vi "(Pop-up) Header Make.vi"(7 "IN Info":string, 8 "error in (no error)":errorcluster caption="에러 입력(에러 없음)", 9 "IN RB/GB":bool, 10 "IN Current Limit":dbl format="%.2f mA", 11 "IN Taget Voltage":dbl format="%.1f V") -> (0 "error out":errorcluster caption="에러 출력", 1 "Start":bool, 2 "Out Start Delay":dbl format="%<%H:%M:%S>t")   [LabVIEW 2017]
uses:
  <vilib>/Utility/miscctls.llb/LVPointTypeDef.ctl
panel:
  in  "Start Delay":dbl format="%<%H:%M:%S>t"
  out "RB/GB":bool
  out "Init":bool
  in  "Apply":bool
  out "Current Limit":dbl format="%.2f mA"
  out "Taget Voltage":dbl format="%.1f V"
  out "Info":string
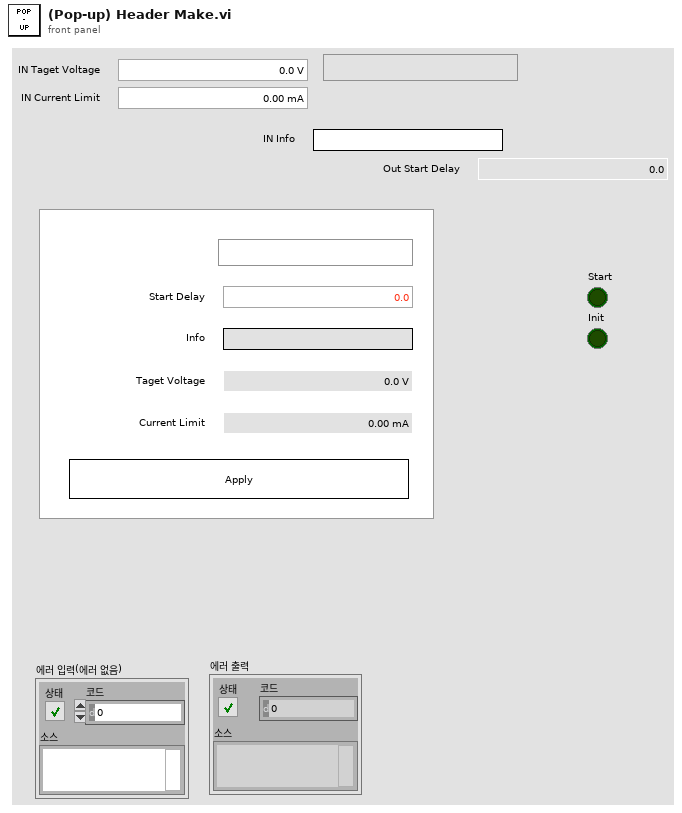
[diagram p1: front panel]
types:
  T1 = typedef "LVPointTypeDef.ctl" = cluster{"Horizontal":i16, "Vertical":i16}
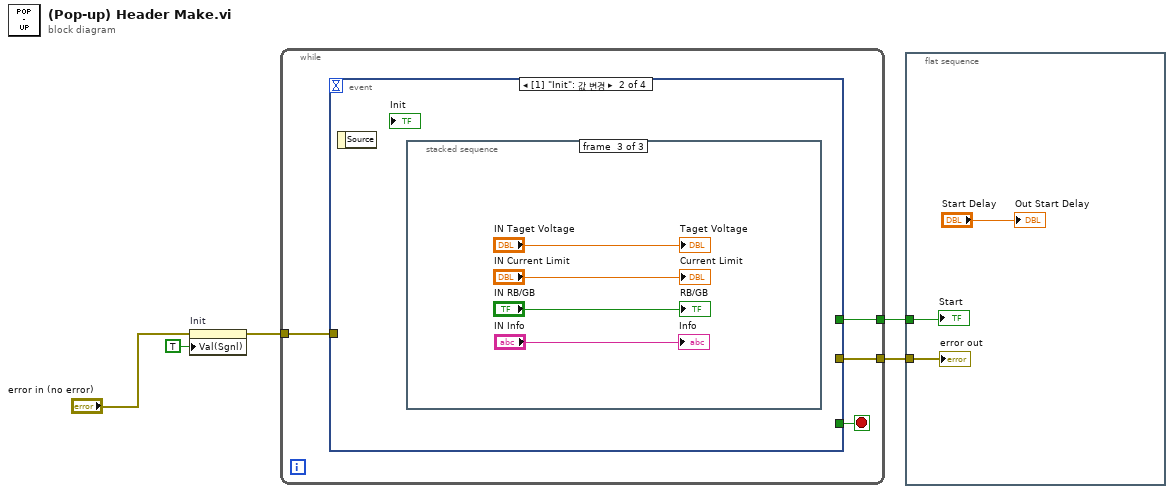
[diagram p0: block diagram]
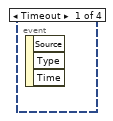
[diagram p2: hidden frame]
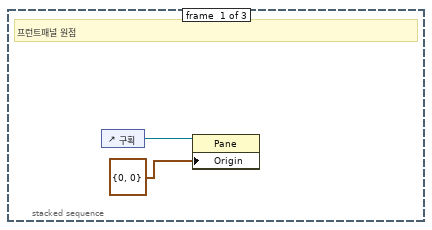
[diagram p3: hidden frame]
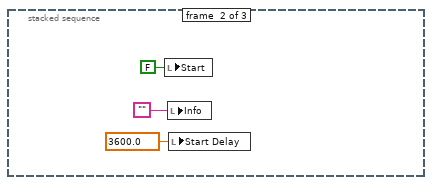
[diagram p4: hidden frame]
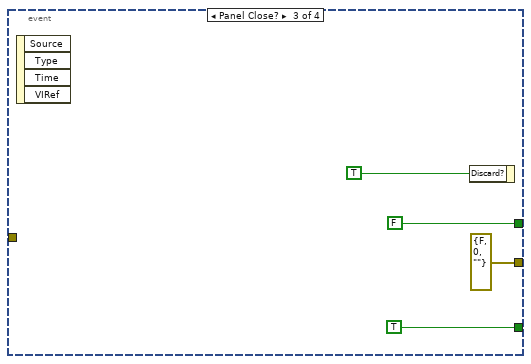
[diagram p5: hidden frame]
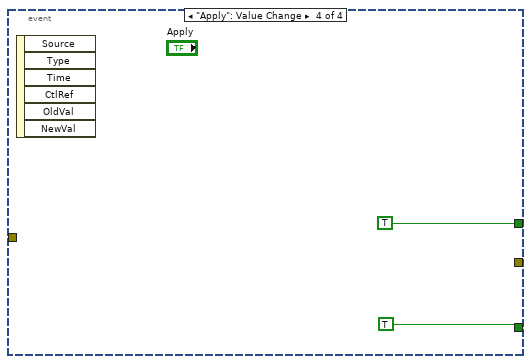
[diagram p6: hidden frame]
diagram:
  n1 = property on="Init" class="Bool (엄격한)"(error in="error in (no error)", "Val(Sgnl)"=TRUE ("값(신호)")) -> (error out=w2:errorcluster)  [unwired: 1 in, 1 out]
  n2 = while {
    tunnel: [w8] -> w5
    tunnel: w2 -> [w7]
    tunnel: [w6] -> w1
    stop <- w9 stop-if-true
    n3 = event shown="[1] \"Init\": 값 변경" {
      selector: _ -> [_ _ _ _]
      dyn-events: _ -> [_ _ _ _]
      timeout: _ -> [_ _ _ _]
      tunnel: [_ _ TRUE TRUE] -> w9
      tunnel: [_ _ FALSE TRUE] -> w8
      tunnel: w7 -> [_ _ _ _]
      tunnel: [_ _ errorcluster {"status"=FALSE, "code"=0, "source"=""} ("에러 상수") _] -> w6
      event Timeout {
        n4 = event-data() -> ()  [unwired: 1 in, 3 out]
      }
      event "Init": Value Change {
        n5 = event-data() -> ()  [unwired: 1 in, 1 out]
        n6 = stacked-sequence {
          frame #0 {
            # "프런트패널 원점"
            n7 = control-ref of="구획"() -> (w11:refnum<vi>)
            n8 = property class="Pane"(reference=w11, "Origin"=T1 {"Horizontal"=0, "Vertical"=0} ("원점")) -> ()  [unwired: 1 in, 2 out]
          }
          frame #1 {
            n9 = local write "Start"(FALSE ("Start")) -> ()
            n10 = local write "Info"("") -> ()
            n11 = local write "Start Delay"(3600.0 ("Start Delay")) -> ()
          }
          frame #2 {
            "Taget Voltage" <- "IN Taget Voltage"
            "Current Limit" <- "IN Current Limit"
            "RB/GB" <- "IN RB/GB"
            "Info" <- "IN Info"
          }
        }
      }
      event Panel Close? {
        n12 = event-data() -> ()  [unwired: 1 in, 4 out]
        n13 = event-data("Discard?"=TRUE) -> ()  [unwired: 1 in, 1 out]
      }
      event "Apply": Value Change {
        n14 = event-data() -> ()  [unwired: 1 in, 6 out]
      }
    }
  }
  n15 = flat-sequence {
    tunnel: w5 -> [w27]
    tunnel: w1 -> [w26]
    frame #0 {
      "error out" <- w26
      "Start" <- w27
      "Out Start Delay" <- "Start Delay"
    }
  }
